vi "Read IConfigure.vi"(8 "error in (no error)":errorcluster, 11 "Thermometer Base in":refnum<class "Thermometer Base.lvclass">) -> (0 "error out":errorcluster, 2 "IConfigure":refnum<class "IConfigure.lvclass">, 3 "Thermometer Base out":refnum<class "Thermometer Base.lvclass">)   [LabVIEW 2023, in "Thermometer.lvlib" / "Thermometer Base.lvlib" / "Thermometer Base.lvclass"]
uses:
  Thermometer Base.lvclass
  Interfaces/IConfigure/IConfigure.lvclass
  Thermometer Base.lvclass/Thermometer Base.ctl
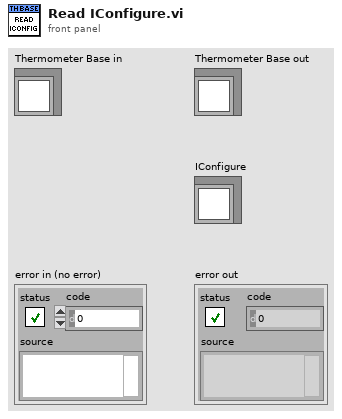
[diagram p1: front panel]
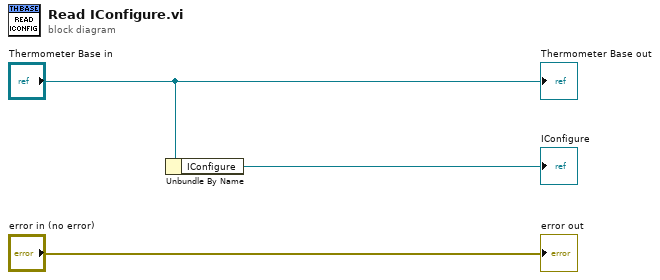
[diagram p0: block diagram]
diagram:
  n1 = Unbundle By Name("Thermometer Base in") -> ("IConfigure"=→"IConfigure":refnum<class "IConfigure.lvclass">)
  "error out" <- "error in (no error)"
  "Thermometer Base out" <- "Thermometer Base in"
